vi "autothreshold.vi"(0 "MCS_bg_corr":sgl[](array[numeric]), 1 "Parameters in":T1, 2 "automatic threshold":bool, 3 "x * sigma":u8=3, 4 "# bins":i32=55) -> (5 "Parameters out":T1, 6 "Intensity Historgram":cluster{"Axis":dbl[], "Histogram":i32[]}(graph), 7 "mean, std.dev":dbl[](array[numeric]) format="%.2f")   [LabVIEW 2009]
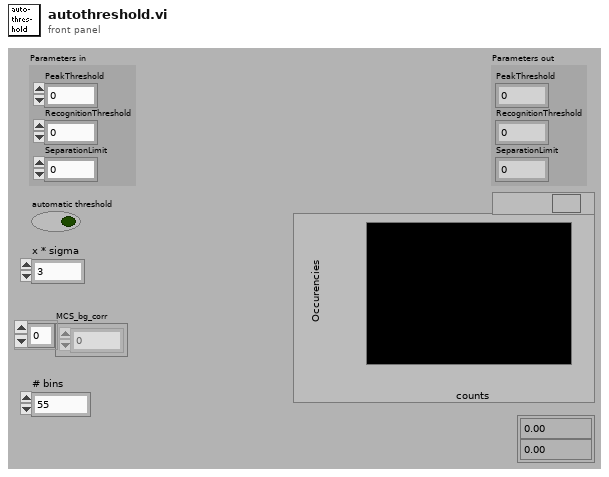
[diagram p1: front panel]
types:
  T1 = cluster{"PeakThreshold":u32, "RecognitionThreshold":u32, "SeparationLimit":sgl}
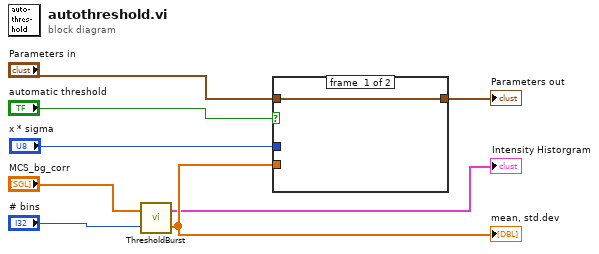
[diagram p0: block diagram]
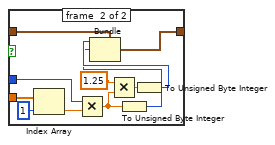
[diagram p2: hidden frame]
diagram:
  n1 = call "ThresholdBurst.vi"("# bins"="# bins", "Array"="MCS_bg_corr") -> ("Best Fit Coefficients"=w3:dbl[], "Intensity-Histogram"=→"Intensity Historgram":cluster{"Axis":dbl[], "Histogram":i32[]})
  "mean, std.dev" <- w3
  n2 = case shown="True" "automatic threshold" {
    tunnel: "x * sigma" -> [_ w19]
    tunnel: w3 -> [_ w17]
    tunnel: "Parameters in" -> [w9 w15]
    tunnel: [w9 w14] -> w7
    frame #0 {
    }
    frame #1 {
      n3 = Index Array(array=w17, index=1) -> (element=w20:dbl)
      n4 = Multiply(x=w19, y=w20) -> (x*y=w13:dbl)
      n5 = Multiply(x=1.25, y=w13) -> (x*y=w12:dbl)
      n6 = To Unsigned Byte Integer(number=w13) -> (unsigned 8bit integer=w10:u8)
      n7 = To Unsigned Byte Integer(number=w12) -> (unsigned 8bit integer=w11:u8)
      n8 = Bundle(cluster=w15, "PeakThreshold"=w11, "RecognitionThreshold"=w10) -> (w14:T1)  [unwired: 1 in]
    }
  }
  "Parameters out" <- w7
